vi "Get Deployment Target.vi"(8 "error in (no error)":errorcluster) -> (0 "error out":errorcluster, 3 "deployment_target":string)   [LabVIEW 2021, in "NI Discovery V1 Client.lvlib"]
uses:
  NI Discovery V1 Client.lvlib
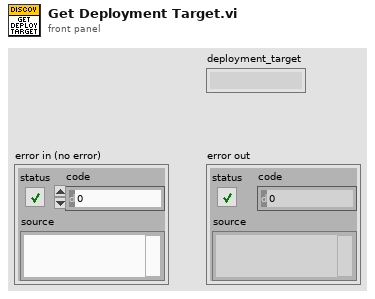
[diagram p1: front panel]
types:
  T1 = typedef "ni.measurementlink.discovery.v1.api.lvlib/ni_measurementlink_discovery_v1_EnumerateComputeNodesResponse.ctl" = cluster{"compute_nodes":T2[]}
  T2 = typedef "ni.measurementlink.discovery.v1.api.lvlib/ni_measurementlink_discovery_v1_ComputeNodeDescriptor.ctl" = cluster{"url":string, "is_local":bool}
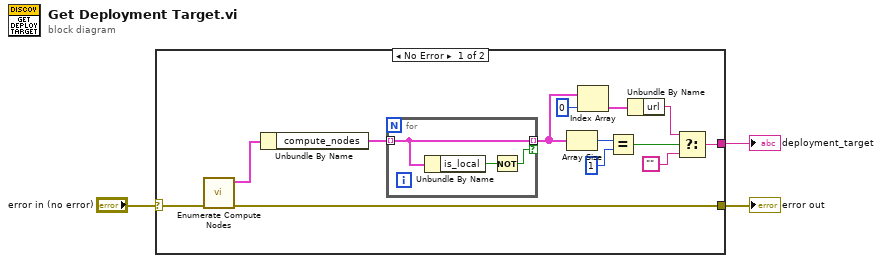
[diagram p0: block diagram]
diagram:
  n1 = case shown="No Error" "error in (no error)" {
    selector: "error in (no error)" -> [w4 w20]
    tunnel: [w16 _] -> w3
    tunnel: [w5 w20] -> w2
    frame No Error {
      n2 = call "Enumerate Compute Nodes.vi"("error in"=w4) -> ("error out"=w5:errorcluster, "response data"=w6:T1)  [unwired: 9 in]
      n3 = Unbundle By Name(w6) -> ("compute_nodes"=w7:T2[])
      n4 = for {
        tunnel: w7 -> [w19] mode=indexing
        tunnel: [w19] -> w10 mode=indexing if=w18
        n5 = Unbundle By Name(w19) -> ("is_local"=w17:bool)
        n6 = Not(x=w17) -> (.not. x?=w18:bool)
      }
      n7 = Array Size(array=w10) -> (size(s)=w8:i32)
      n8 = Index Array(array=w10, index=0) -> (element=w12:T2)
      n9 = Equal?(x=w8, y=1) -> (x = y?=w13:bool)
      n10 = Unbundle By Name(w12) -> ("url"=w14:string)
      n11 = Select(t=w14, s=w13, f="") -> (s? t:f=w16:string)
    }
    frame Error {
    }
  }
  "deployment_target" <- w3
  "error out" <- w2
